vi "Parse TSA Report File.vi"(8 "error in (no error)":errorcluster, 11 "TSA Report File Path":path) -> (0 "error out":errorcluster, 2 "TSA Errors as Plain Text":string, 3 "TSA Messages[]":T1[](array[typedef]))   [LabVIEW 2016, in "SLL TestStand.lvlib"]
uses:
  SLL TestStand.lvlib
  _Typedefs/TSA Error Message Cluster.ctl
  SLL File IO/XML/_SubVIs/Initialize XML from File.vi
  SLL File IO/XML/_SubVIs/Get XPath Text.vi
  SLL File IO/SLL File IO.lvlib
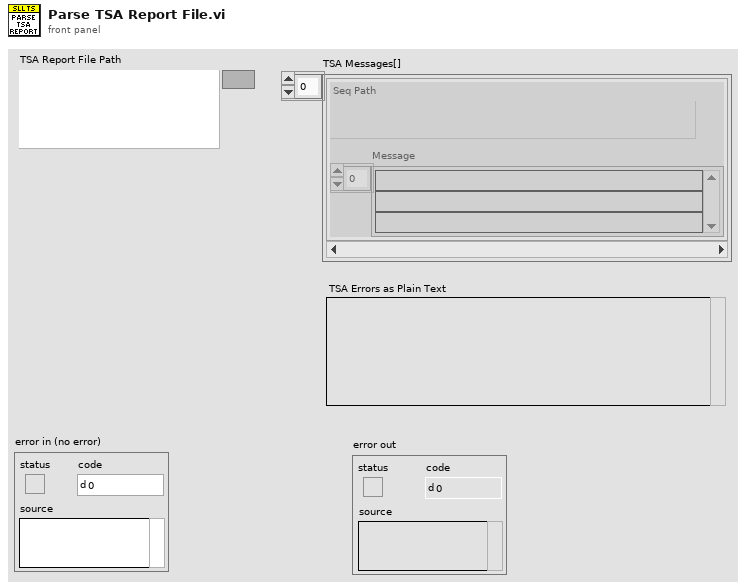
[diagram p1: front panel]
types:
  T1 = typedef "SLL TestStand.lvlib/TSA Error Message Cluster.ctl" = cluster{"Seq Path":path, "Message":string[]}
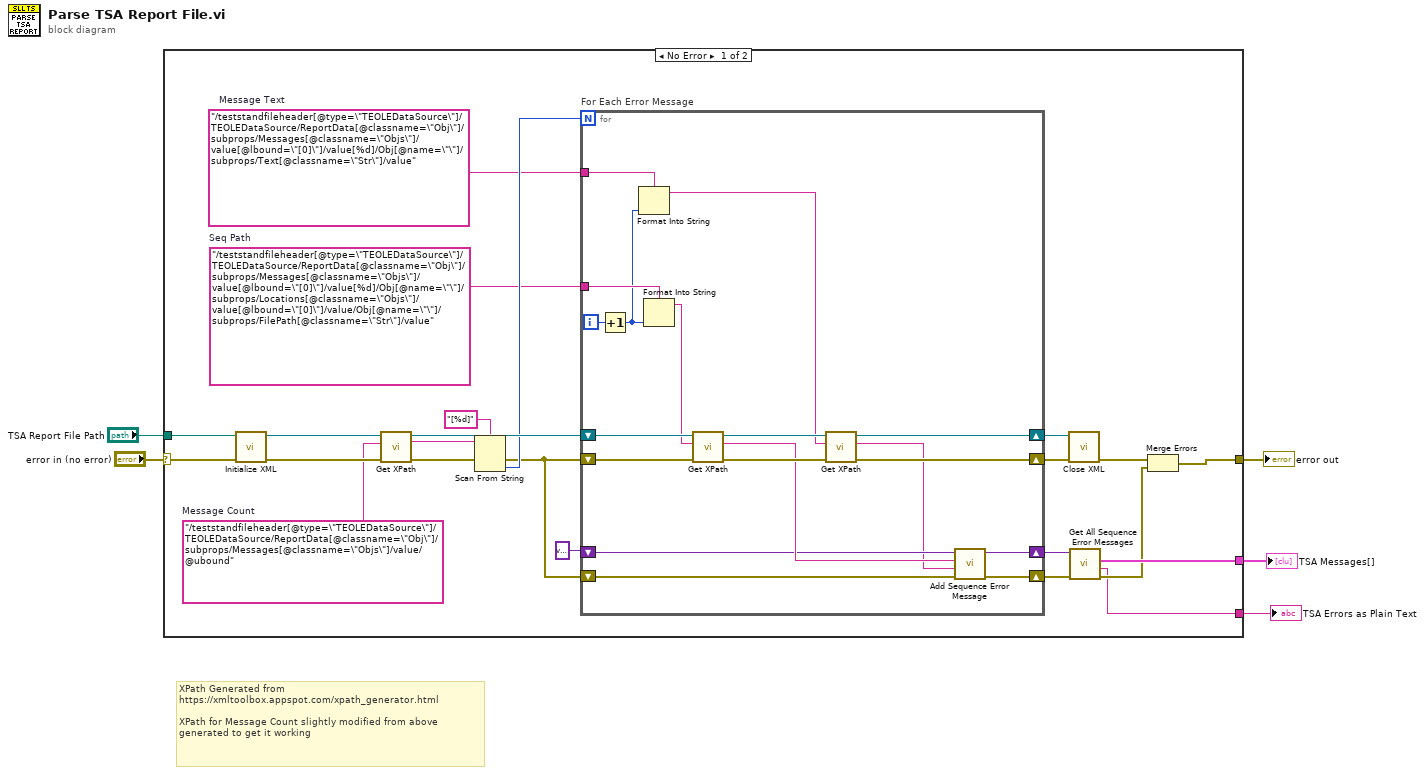
[diagram p0: block diagram]
diagram:
  # "XPath Generated from\nhttps://xmltoolbox.appspot.com/xpath_generator.html\n\nXPath for Message Count slightly modified from above generated to get it working"
  n1 = case shown="No Error" "error in (no error)" {
    selector: "error in (no error)" -> [w28 w47]
    tunnel: [w8 w47] -> w4
    tunnel: "TSA Report File Path" -> [w26 _]
    tunnel: [w11 _] -> w2
    tunnel: [w6 _] -> w1
    frame No Error {
      w14 = "/teststandfileheader[@type=\"TEOLEDataSource\"]/TEOLEDataSource/ReportData[@classname=\"Obj\"]/subprops/Messages[@classname=\"Objs\"]/value[@lbound=\"[0]\"]/value[%d]/Obj[@name=\"\"]/subprops/Text[@classname=\"Str\"]/value"  # Message Text
      w13 = "/teststandfileheader[@type=\"TEOLEDataSource\"]/TEOLEDataSource/ReportData[@classname=\"Obj\"]/subprops/Messages[@classname=\"Objs\"]/value[@lbound=\"[0]\"]/value[%d]/Obj[@name=\"\"]/subprops/Locations[@classname=\"Objs\"]/value[@lbound=\"[0]\"]/value/Obj[@name=\"\"]/subprops/FilePath[@classname=\"Str\"]/value"  # Seq Path
      w23 = "/teststandfileheader[@type=\"TEOLEDataSource\"]/TEOLEDataSource/ReportData[@classname=\"Obj\"]/subprops/Messages[@classname=\"Objs\"]/value/@ubound"  # Message Count
      n2 = call-poly "Initialize XML.vi"("error in (no error)"=w28, "XML File Path"=w26) -> ("error out"=w27:errorcluster, "DOM document out"=w24:refnum<k20>)  [unwired: 8 in]
      n3 = call-poly "Get XPath.vi"("error in (no error)"=w27, "XPath Expression"=w23, "DOM document in"=w24) -> ("error out"=w25:errorcluster, "Node Text"=w18:string, "DOM document out"=w21:refnum<k20>)  [unwired: 5 in, 1 out]
      n4 = Scan From String(format string="[%d]", input string=w18, error in=w25) -> (error out=w10:errorcluster, output 1=w16:i32)  [unwired: 2 in, 2 out]
      n5 = for "For Each Error Message" {
        N: w16 -> [_]
        shift-right: [w39] -> w22
        shift-left: w10 -> [w46]
        shift-right: [w37] -> w19
        shift-left: w21 -> [w44]
        tunnel: w13 -> [w43]
        tunnel: w14 -> [w42]
        shift-right: [w33] -> w12
        shift-left: variant -> [w32]
        shift-right: [w30] -> w9
        shift-left: w10 -> [w29]
        i -> [w41]
        n6 = Increment(x=w41) -> (x+1=w35:i32)
        n7 = Format Into String(format string=w42, w35) -> (resulting string=w36:string)  [unwired: 2 in, 1 out]
        n8 = Format Into String(format string=w43, w35) -> (resulting string=w40:string)  [unwired: 2 in, 1 out]
        n9 = call-poly "Get XPath.vi"("error in (no error)"=w46, "XPath Expression"=w40, "DOM document in"=w44) -> ("error out"=w45:errorcluster, "Node Text"=w34:string, "DOM document out"=w38:refnum<k20>)  [unwired: 5 in, 1 out]
        n10 = call-poly "Get XPath.vi"("error in (no error)"=w45, "XPath Expression"=w36, "DOM document in"=w38) -> ("error out"=w39:errorcluster, "Node Text"=w31:string, "DOM document out"=w37:refnum<k20>)  [unwired: 5 in, 1 out]
        n11 = call "Add Sequence Error Message.vi"("error in (no error)"=w29, "Msg"=w31, "Seq Path"=w34, "Variant in"=w32) -> ("error out"=w30:errorcluster, "Variant out"=w33:variant)  [unwired: 6 in]
      }
      n12 = call "Close XML.vi"("error in (no error)"=w22, "DOM document in"=w19) -> ("error out"=w20:errorcluster)  [unwired: 9 in]
      n13 = call "Get All Sequence Error Messages.vi"("error in (no error)"=w9, "Variant in"=w12) -> ("error out"=w7:errorcluster, "TSA Errors as Plain Text"=w6:string, "TSA Errors[]"=w11:T1[])  [unwired: 6 in, 1 out]
      n14 = Merge Errors(w20, w7) -> (w8:errorcluster)
    }
    frame Error {
    }
  }
  "error out" <- w4
  "TSA Messages[]" <- w2
  "TSA Errors as Plain Text" <- w1
